vi "stop.vi"(8 "error in (no error)":errorcluster, 11 "Counter in":refnum<class "Counter.lvclass">) -> (0 "error out":errorcluster, 3 "Counter out":refnum<class "Counter.lvclass">)   [LabVIEW 2014, in "Counter.lvclass"]
uses:
  Counter.lvclass
  Counter.lvclass/Counter.ctl
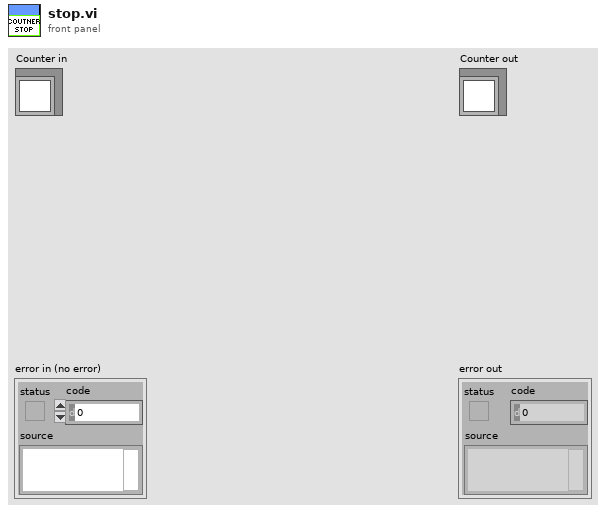
[diagram p1: front panel]
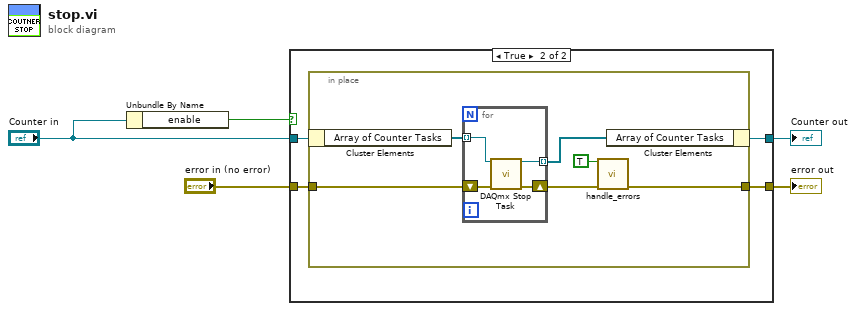
[diagram p0: block diagram]
diagram:
  n1 = Unbundle By Name("Counter in") -> ("enable"=w1:bool)
  n2 = case shown="True" w1 {
    tunnel: [w7 w11] -> w4
    tunnel: "error in (no error)" -> [w7 w10]
    tunnel: "Counter in" -> [w6 w9]
    tunnel: [w6 w8] -> w2
    frame False {
    }
    frame True {
      n3 = in-place {
        in-place-border: [w13] -> w11
        in-place-border: w10 -> [w17]
        n4 = in-place-cluster #1(w9) -> ("Array of Counter Tasks"=w16:refnum<k21>[])
        n5 = for {
          tunnel: w16 -> [w21] mode=indexing
          shift-right: [w19] -> w14
          shift-left: w17 -> [w20]
          tunnel: [w18] -> w15 mode=indexing
          n6 = call <vilib>:"DAQmx Stop Task.vi"("task/channels in"=w21, "error in"=w20) -> ("task out"=w18:refnum<k21>, "error out"=w19:errorcluster)  [unwired: 12 in]
        }
        n7 = call "handle_errors.vi"("Exit Operation"=TRUE ("Exit Measurement"), "error in (no error)"=w14) -> ("error out"=w13:errorcluster)  [unwired: 13 in]
        n8 = in-place-cluster #1("Array of Counter Tasks"=w15) -> (w8:refnum<class "Counter.lvclass">)
      }
    }
  }
  "error out" <- w4
  "Counter out" <- w2
